vi "Check Buffer Size (1B).vi"(5 "source vi name":string, 7 "bytes to move":u64 format="%d bytes", 8 "error in (no error)":errorcluster, 9 "offset (0)":u64 format="%d bytes", 10 "buffer count":u64 format="%d elements", 11 "Pointer in":refnum<class "Pointer.lvclass">) -> (0 "error out":errorcluster, 1 "offset":u64 format="%d bytes", 2 "buffer count":u64 format="%d elements", 3 "Pointer out":refnum<class "Pointer.lvclass">)   [LabVIEW 2017, in "Memory Manager.lvlib" / "Pointer.lvclass"]
uses:
  Pointer.lvclass
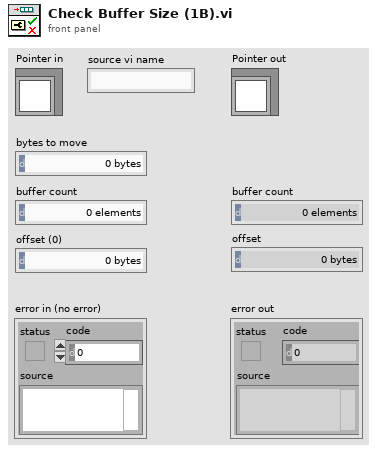
[diagram p1: front panel]
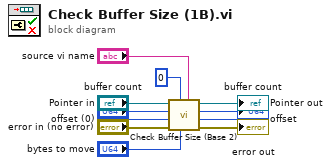
[diagram p0: block diagram]
diagram:
  n1 = call "Check Buffer Size (Base 2).vi"("source vi name"="source vi name", "bytes to move"="bytes to move", "power of 2"=i16 0, "error in (no error)"="error in (no error)", "offset (0)"="offset (0)", "buffer count"="buffer count", "Pointer in"="Pointer in") -> ("error out"=→"error out":errorcluster, "offset"=→"offset":u64, "buffer count"=→"buffer count":u64, "Pointer out"=→"Pointer out":refnum<class "Pointer.lvclass">)  [unwired: 1 in]
